vi "Test Listen.vi"() -> ()   [LabVIEW 2013]
panel:
  out "error IO":errorcluster
  out "data out":string
  in  "stop":bool
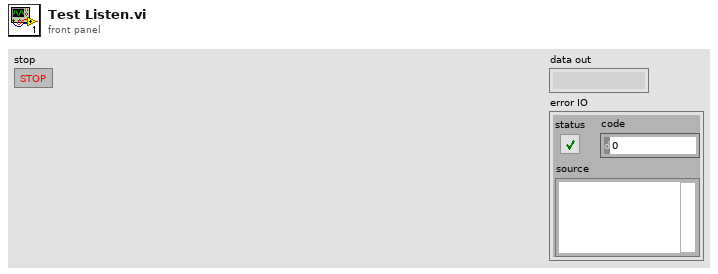
[diagram p1: front panel]
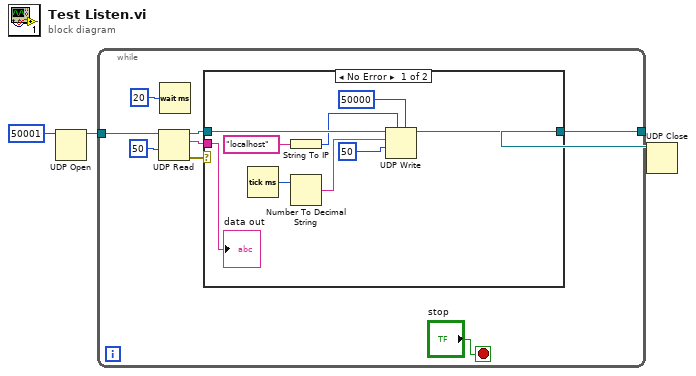
[diagram p0: block diagram]
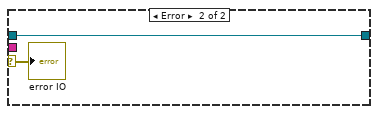
[diagram p2: hidden frame]
diagram:
  n1 = UDP Open(11:u16 50001 ("port")) -> (port=w2:refnum<k16>)  [unwired: 4 in, 2 out]
  n2 = while {
    tunnel: w2 -> [w9]
    tunnel: [w4] -> w1
    stop <- "stop" stop-if-true
    n3 = UDP Read(connection ID=w9, timeout ms (25000)=50) -> (data out=w7:string, error out=w8:errorcluster, 3:w6:refnum<k16>)  [unwired: 2 in, 2 out]
    n4 = Wait (ms)(milliseconds to wait=u32 20) -> ()  [unwired: 1 out]
    n5 = case shown="No Error" w8 {
      selector: w8 -> [_ w22]
      tunnel: w7 -> [w20 _]
      tunnel: w6 -> [w19 w21]
      tunnel: [w12 w21] -> w4
      frame No Error {
        n6 = Tick Count (ms)() -> (millisecond timer value=w15:u32)
        n7 = String To IP(1:"localhost") -> (0:w17:u32)
        n8 = Number To Decimal String(number=w15) -> (decimal integer string=w14:string)  [unwired: 1 in]
        n9 = UDP Write(address=w17, port or service name=u16 50000, connection ID=w19, data in=w14, 9:50 ("timeout ms (25000)")) -> (3:w12:refnum<k16>)  [unwired: 1 in, 1 out]
        "data out" <- w20
      }
      frame Error {
        "error IO" <- w22
      }
    }
  }
  n10 = UDP Close(connection ID=w1) -> ()  [unwired: 1 in, 2 out]
